vi "GoldenHour.vi"() -> ()   [LabVIEW 2019]
doc: "This example demonstrates how to read X, Y, and Z accelerations using the MMA8452 accelerometer."
uses:
  <vilib>/userdefined/High Color/IMAQdx.ctl
  System.Windows.Forms
  <vilib>/Utility/miscctls.llb/LVForegroundBackgroundColorsTypeDef.ctl
  <vilib>/Instr/_visa.llb/VISA Configure Serial Port (Instr).vi
  <vilib>/MakerHub/LINX/Public/Utilities/Open Serial.vi
  <vilib>/Utility/file.llb/Write Delimited Spreadsheet (DBL).vi
  <vilib>/Utility/file.llb/Read Delimited Spreadsheet (DBL).vi
  <vilib>/MakerHub/LINX/LMH-LINX.lvlib
  <vilib>/MakerHub/LINX/Public/Sensors/Accelerometer/MMA8452/MMA8452.lvlib
  <vilib>/vision/driver/NI_Vision_Acquisition_Software.lvlib
panel:
  in  "file path (dialog if empty)":path caption="파일 경로(비었을 경우 대화 상자 창)"
  in  "경로 2":path=path "C:/Users/suit9/Documents/카카오톡 받은 파일/inventors.csv"
  in  "경로":path=path "C:/Users/suit9/Documents/카카오톡 받은 파일/inventors - 복사본.csv"
  in  "A Port":refnum<visa-resource-name>
  in  "B Port":refnum<visa-resource-name>
  in  "Camera":T1
  in  "Grbl":refnum<visa-resource-name>="COM5"
  in  "B 설비 이상":bool
  in  "A 설비 이상":bool
  in  "B_stop":bool
  in  "A_stop":bool
  in  "CAM_stop":bool
  in  "P_stop":bool
  in  "I2C Channel 2":u8
  in  "CAM_Control":T2
  in  "Page_B":bool
  in  "Page_A":bool
  in  "Page_ALL":bool
  in  "distance(mm)":dbl=4.0
  out "Y_FFT 2":dbl[](graph)
  out "Z_FFT 2":dbl[](graph)
  in  "B_X_그림":path=path "C:/Users/suit9/Desktop/대회준비 모든파일/슈퍼이상.png"
  in  "A_X_그림":path=path "C:/Users/suit9/Desktop/대회준비 모든파일/정상.png"
  in  "B_Z":path=path "C:/Users/suit9/Desktop/대회준비 모든파일/엑셀모음/B_Z.csv"
  in  "B_Y":path=path "C:/Users/suit9/Desktop/대회준비 모든파일/엑셀모음/B_Y.csv"
  in  "B_X":path=path "C:/Users/suit9/Desktop/대회준비 모든파일/엑셀모음/B_X.csv"
  in  "A_Z":path=path "C:/Users/suit9/Desktop/대회준비 모든파일/엑셀모음/A_Z.csv"
  in  "A_Y":path=path "C:/Users/suit9/Desktop/대회준비 모든파일/엑셀모음/A_Y.csv"
  in  "A_X":path=path "C:/Users/suit9/Desktop/대회준비 모든파일/엑셀모음/A_X.csv"
  in  "dist(mm)":dbl
  in  "dist(mm) 2":dbl
  in  "A설비":dbl
  in  "B설비":dbl
  out "MoveString 5":string
  out "MoveString 4":string
  out "number 2":dbl format="%.2f"
  out "MoveString 3":string
  out "Version":string
  out "Connecting to":string
  in  "Send G-code":bool
  in  "Select G-code file":bool
  out "G-code list":string
  in  "Local-Home":bool
  in  "Pos Button":bool
  out "Local-Pos":cluster{"X":dbl, "Y":dbl, "Z":dbl}
  out "M-Pos":cluster{"X":dbl, "Y":dbl, "Z":dbl}
  in  "Machine-Home":bool
  in  "Send":bool
  in  "One line Command":string
  in  "SetLocal":bool
  out "Local Origin":cluster{"X":dbl, "Y":dbl, "Z":dbl}
  out "MoveString":string
  out "MoveString 2":string
  out "Command":string
  out "History":string
  out "Response":string
  in  "탭 컨트롤":enum32{"ALL", "A", "B"}(tab)
  out "특이사항":string="A설비 이상진동 다량발생 확인요함\n\n설비 이력\n\n# 이전 A설비 교체 : 2020-09-10\n\n# 이전 B설비 교체 : 2020-08-20\n\n\n"
  out "Boolean Rectangle 3":bool
  out "Boolean Rectangle":bool
  out "Time series 4":T3(graph)
  out "Time series 3":T3(graph)
  out "수명예측":dbl(knob) caption="Gauge" scale=0.1..100.0
  out "CAM":T4(plugin-control)
  out "all rows":dbl[][](array[numeric]) caption="NUM(A)    LOSS     THR        Vib"
  out "수명예측":dbl(knob) caption="Gauge" scale=0.0..100.0
  out "all rows 2":dbl[][](array[numeric]) caption="NUM(B)        LOSS      THR        Vib"
  out "수명예측":dbl(knob) caption="Gauge" scale=0.0..100.0
  out "문자열 2":string="A : 양호\n\nB : 약간불량, 장시간 운전 허용\n\nC : 불량, 단 시간 운전 허용\n\nD : 극도 불량, 허용불가"
  out "클러스터 6":cluster{"A":bool, "B":bool, "C":bool, "D":bool}
  out "FFT A":dbl[](graph)
  out "Time series A":T3(graph)
  out "CAM":T4(plugin-control)
  in  "PictureBox 5":refnum<k24>(container) caption="Anomaly Detection A"
  out "수명예측":dbl(knob) caption="Gauge" scale=0.1..100.0
  out "문자열":string="A : 양호\n\nB : 약간불량, 장시간 운전 허용\n\nC : 불량, 단 시간 운전 허용\n\nD : 극도 불량, 허용불가"
  out "클러스터 5":cluster{"A":bool, "B":bool, "C":bool, "D":bool}
  out "FFT_B":dbl[](graph)
  out "Time series B":T3(graph)
  out "CAM":T4(plugin-control)
  in  "PictureBox 2":refnum<k24>(container) caption="Anomaly Detection B"
  in  "I2C Channel":u8
  # "GOLDEN\n     Hour"
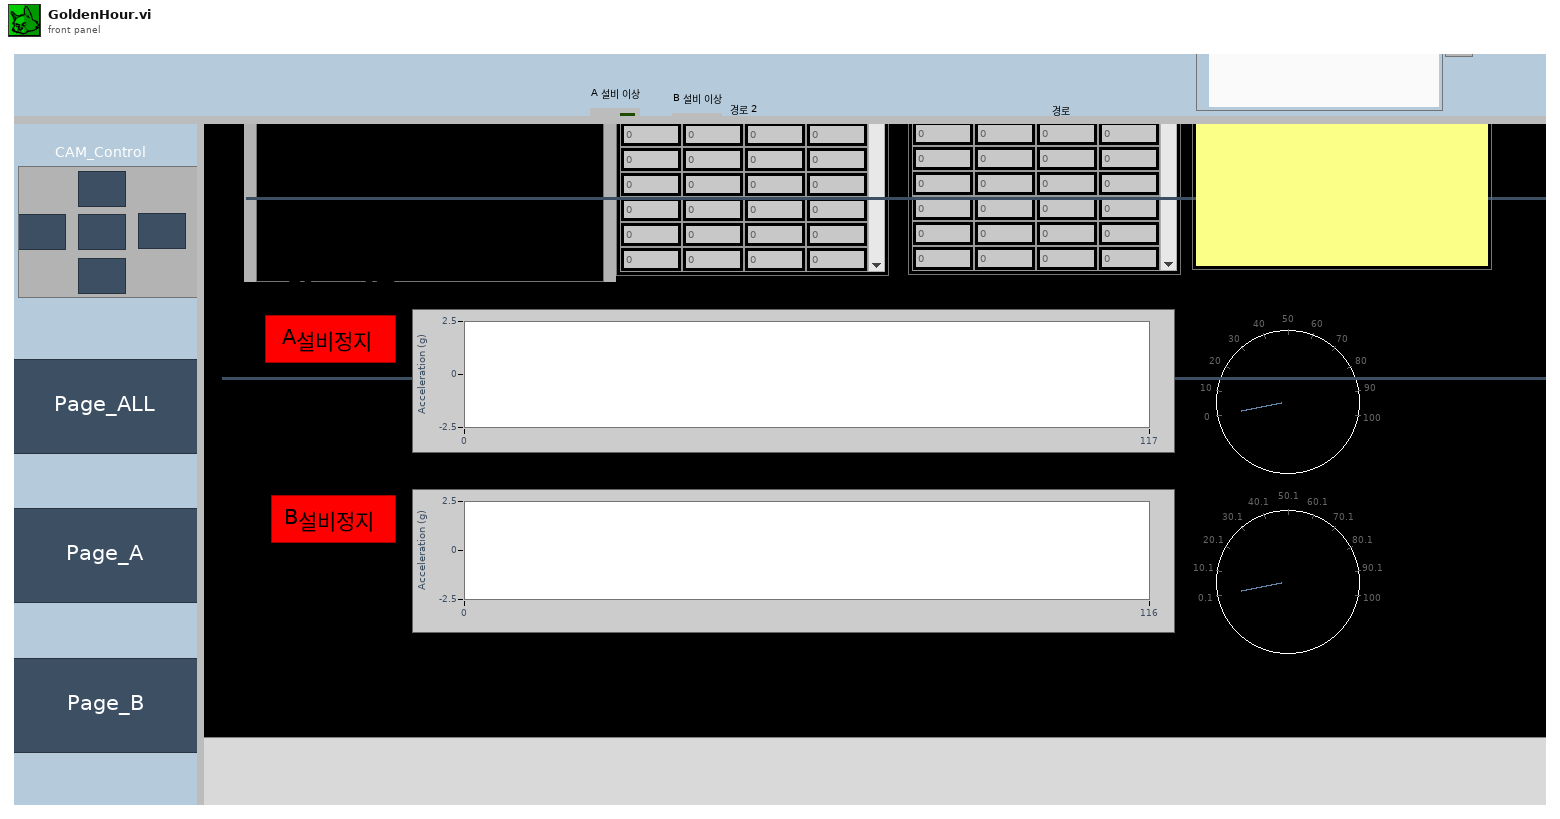
[diagram p1: front panel]
types:
  T1 = typedef "IMAQdx.ctl" = refnum<k21>
  T2 = cluster{"Back Button":bool, "Forward Button":bool, "Up Button":bool, "Down Button":bool, "Reset Button":bool}
  T3 = cluster{"X Axis":dbl, "Y Axis":dbl, "Z Axis":dbl}
  T4 = typedef "IMAQ Image.ctl" = refnum<image>
  T5 = cluster{"VISA resource name":refnum<visa-resource-name>, "baud rate":u32, "data bits":u16, "parity":u16, "stop bits":u16, "flow control":u16}
  T6 = typedef "LVForegroundBackgroundColorsTypeDef.ctl" = cluster{"Foreground Color":u32, "Background Color":u32}
  T7 = typedef "LMH-LINX.lvlib/LINX Ref.ctl" = cluster{"IO":T8, "Interface":T9, "LINX Device Config":T10}
  T8 = typedef "LMH-LINX.lvlib/Platform.ctl" = enum16{"Remote", "Local"}
  T9 = typedef "LMH-LINX.lvlib/Interface.ctl" = enum16{"Serial", "TCP"}
  T10 = typedef "LMH-LINX.lvlib/Device.lvlib/LINX Device Config.ctl" = cluster{"Interface":T9, "COM Port":refnum<visa-resource-name>, "TCP Configuration":T11, "Device Family":u8, "Device ID":u8, "Device Name":string, "TCP Ref":refnum<k5>, "Channels":T12}
  T11 = typedef "LMH-LINX.lvlib/Device.lvlib/TCP Config.ctl" = cluster{"IP Address":string, "Port":u16}
  T12 = typedef "LMH-LINX.lvlib/Channels.ctl" = cluster{"DI":u8[], "DO":u8[], "AI":u8[], "AO":u8[], "PWM":u8[], "QE":u8[], "UART":u8[], "I2C 2":u8[], "SPI":u8[], "CAN":u8[], "Servo":u8[], "AI Ref (V)":dbl, "AI Resolution (Bits)":u8, "AO Ref (V)":dbl, "AO Resolution (Bits)":u8}
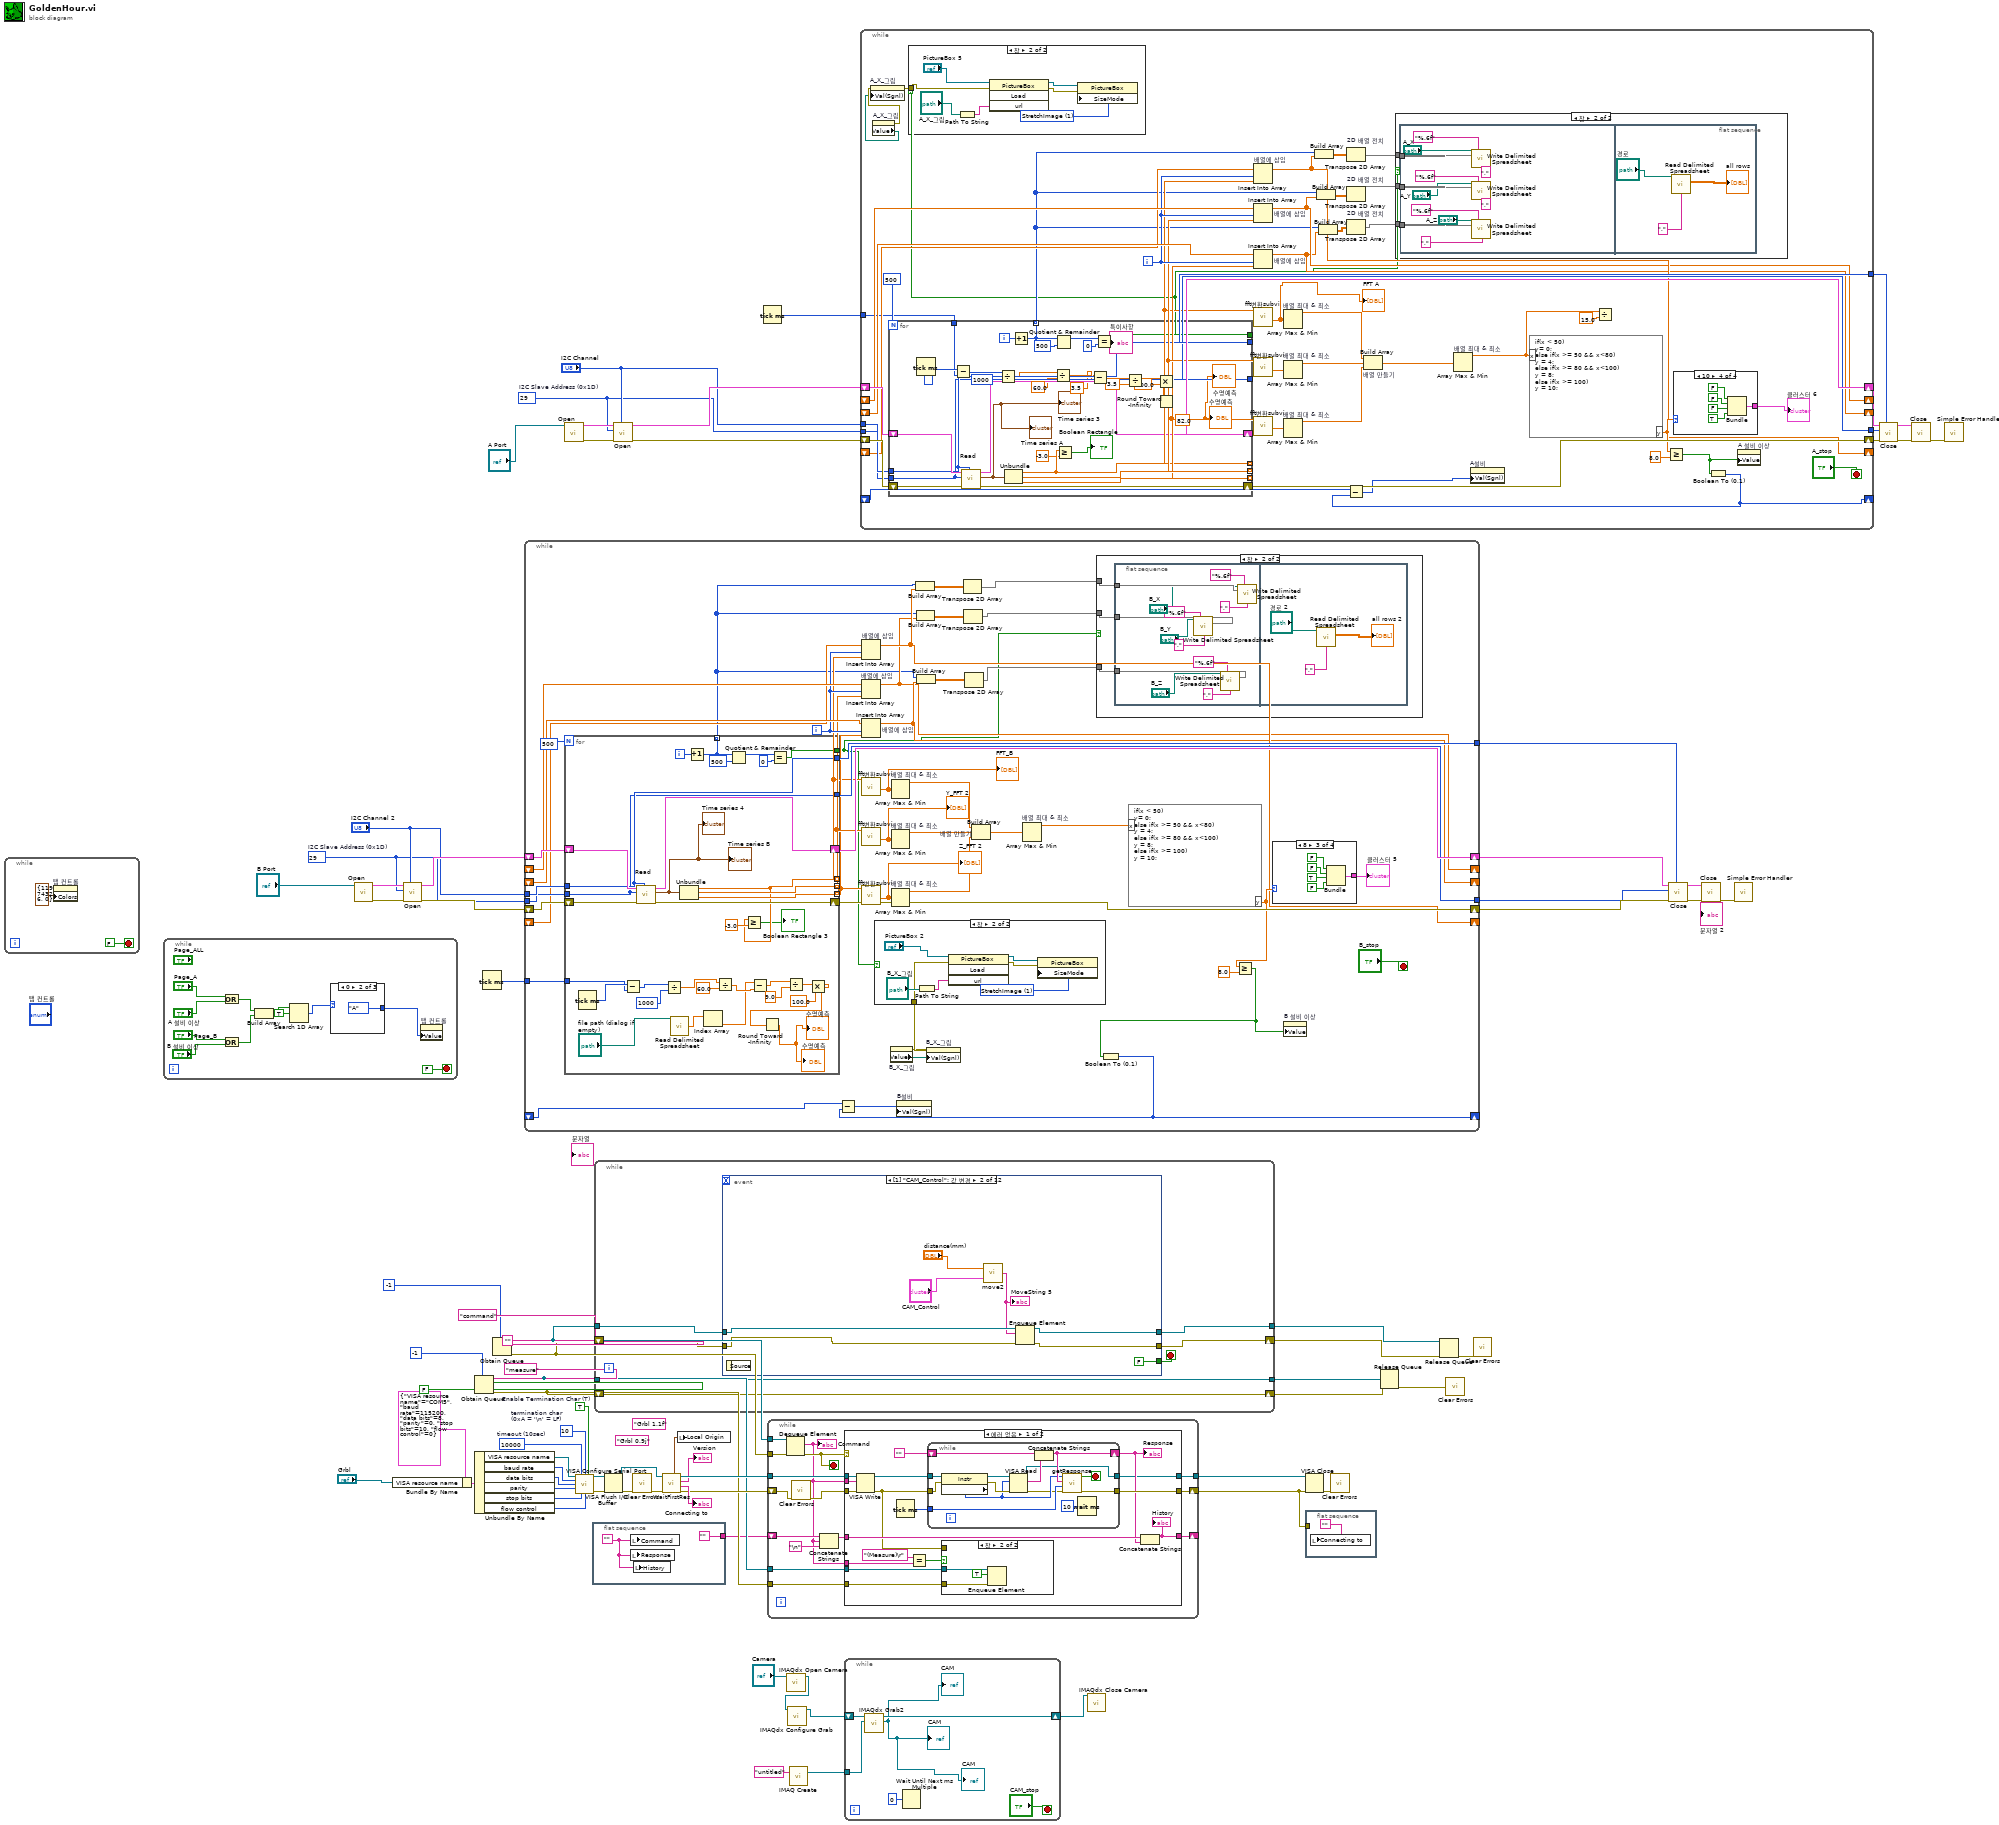
[diagram p0: block diagram]
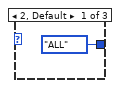
[diagram p2: hidden frame]
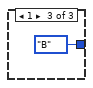
[diagram p3: hidden frame]
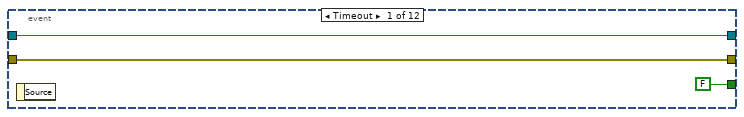
[diagram p4: hidden frame]
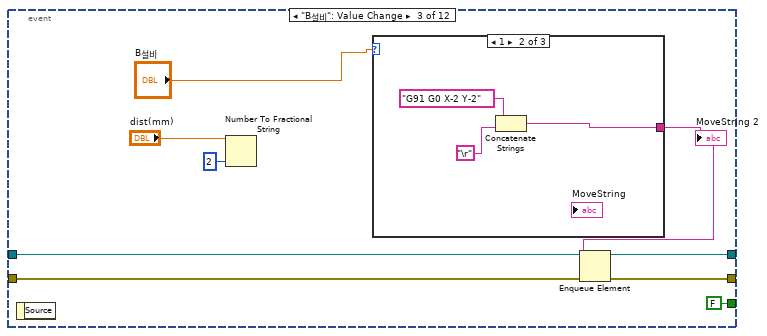
[diagram p5: hidden frame]
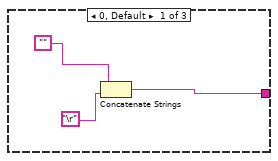
[diagram p6: hidden frame]
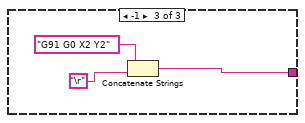
[diagram p7: hidden frame]
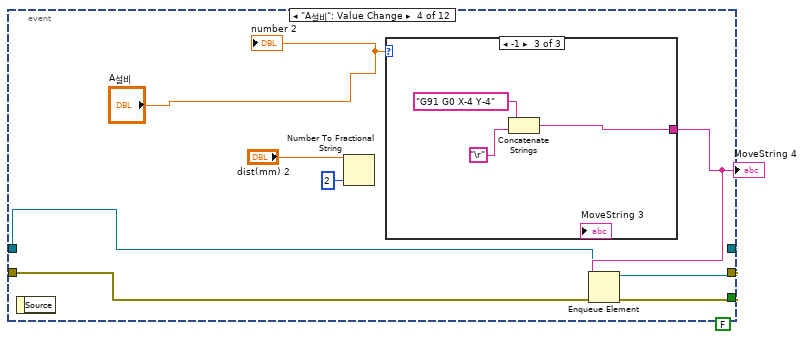
[diagram p8: hidden frame]
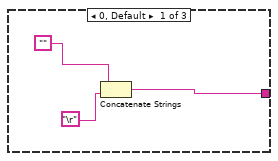
[diagram p9: hidden frame]
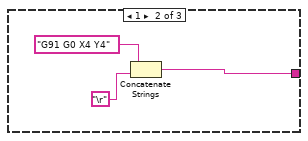
[diagram p10: hidden frame]
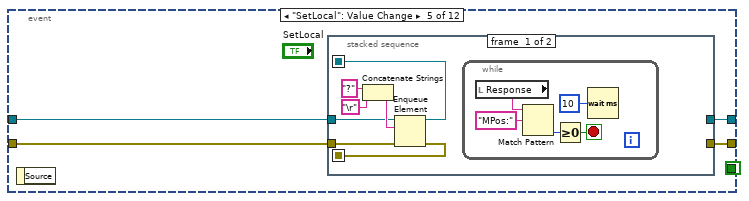
[diagram p11: hidden frame]
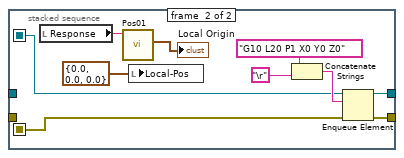
[diagram p12: hidden frame]
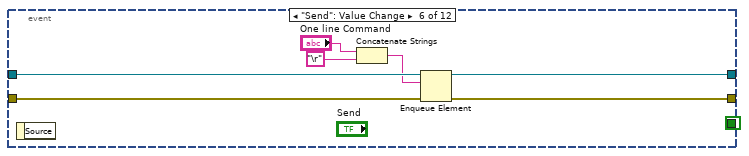
[diagram p13: hidden frame]
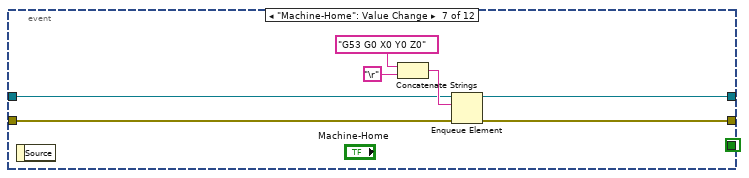
[diagram p14: hidden frame]
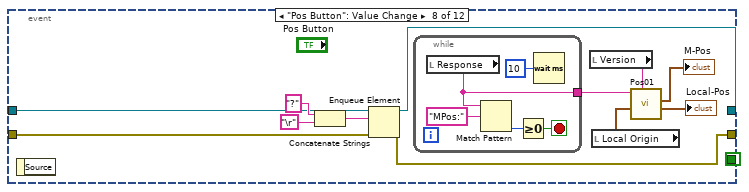
[diagram p15: hidden frame]
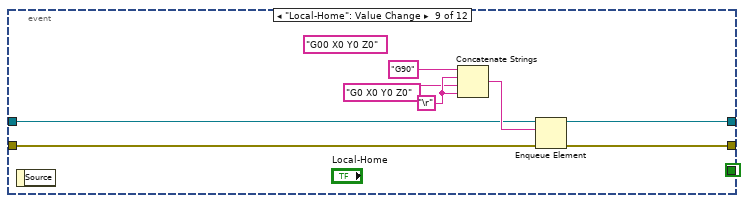
[diagram p16: hidden frame]
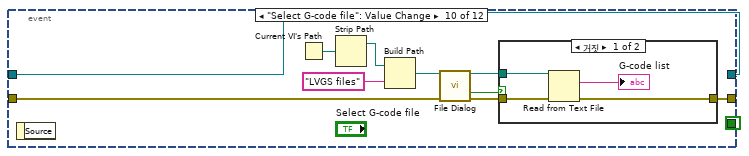
[diagram p17: hidden frame]
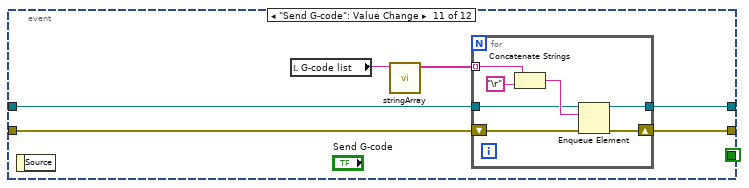
[diagram p19: hidden frame]
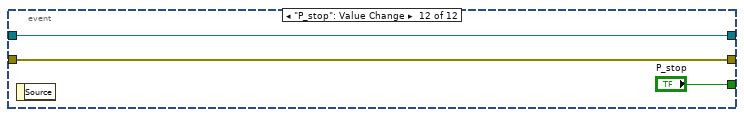
[diagram p20: hidden frame]
diagram:
  (unwired) "Grbl 1.1f" ("Version")
  (unwired) "Grbl 0.9j" ("Version")
  w31 = u8 10  # termination char (0xA = '\n' = LF)
  w42 = TRUE  # Enable Termination Char (T)
  w52 = u32 10000  # timeout (10sec)
  w60 = u8 29  # I2C Slave Address (0x1D)
  w73 = u8 29  # I2C Slave Address (0x1D)
  n1 = while {
    stop <- FALSE stop-if-true
    n2 = property on="탭 컨트롤" class="TabCtl (엄격한)"("Colors"=T6 {"Foreground Color"=11974326, "Background Color"=0} ("색")) -> ()  [unwired: 2 in, 2 out]
  }
  n3 = while {
    stop <- FALSE stop-if-true
    n4 = Or(x="Page_A", y="A 설비 이상") -> (x .or. y?=w87:bool)
    n5 = Or(x="Page_B", y="B 설비 이상") -> (x .or. y?=w86:bool)
    n6 = Build Array(w87, w86) -> (w85:bool[])
    n7 = Search 1D Array(1D array=w85, element=TRUE ("원소")) -> (index of element=w83:i32)  [unwired: 1 in]
    n8 = case shown="0" w83 {
      tunnel: [enum32{"ALL", "A", "B"}."ALL" ("탭 컨트롤") enum32{"ALL", "A", "B"}."A" ("탭 컨트롤") enum32{"ALL", "A", "B"}."B" ("탭 컨트롤")] -> w82
      frame 2, Default {
      }
      frame 0 {
      }
      frame 1 {
      }
    }
    n9 = property on="탭 컨트롤" class="TabCtl (엄격한)"("Value"=w82) -> ()  [unwired: 2 in, 2 out]
  }
  n10 = call-poly <vilib>:"Open.vi"("Serial Port"="B Port") -> ("Error Out"=w65:errorcluster, "LINX Resource"=w64:T7)  [unwired: 8 in, 1 out]
  n11 = Bundle By Name(cluster=T5 {"VISA resource name"="COM5", "baud rate"=115200, "data bits"=8, "parity"=0, "stop bits"=10, "flow control"=0} ("COM"), "VISA resource name"="Grbl") -> (w49:T5)
  n12 = call <vilib>:"Open.vi"("I2C Channel"="I2C Channel 2", "Error In"=w65, "I2C Slave Address (0x1D)"=w60, "LINX Ref"=w64) -> ("Error Out"=w62:errorcluster, "LINX Resource"=w63:T7)  [unwired: 6 in]
  n13 = Obtain Queue(max queue size (-1, unlimited)=-1, name (unnamed)="measure", element data type=FALSE) -> (queue out=w16:refnum<queue>, error out=w15:errorcluster)  [unwired: 2 in, 1 out]
  n14 = Unbundle By Name(w49) -> ("VISA resource name"=w48:refnum<visa-resource-name>, "baud rate"=w47:u32, "data bits"=w46:u16, "parity"=w45:u16, "stop bits"=w44:u16, "flow control"=w43:u16)
  n15 = Tick Count (ms)() -> (millisecond timer value=w1:u32)
  n16 = Obtain Queue(max queue size (-1, unlimited)=-1, name (unnamed)="command", element data type="") -> (queue out=w27:refnum<queue>, error out=w32:errorcluster)  [unwired: 2 in, 1 out]
  n17 = while {
    tunnel: "I2C Channel 2" -> [w139]
    tunnel: w60 -> [w138]
    tunnel: [w135] -> w54
    tunnel: [w134] -> w53
    shift-right: [w136] -> w57
    shift-left: w63 -> [w141]
    shift-right: [w137] -> w58
    shift-left: w62 -> [w140]
    shift-right: [w112] -> _
    shift-left: _ -> [w123]
    shift-right: [w105] -> _
    shift-left: _ -> [w132]
    shift-right: [w106] -> _
    shift-left: _ -> [w131]
    shift-right: [w114] -> _
    shift-left: _ -> [w115]
    tunnel: w1 -> [w99]
    i -> [w129]
    stop <- "B_stop" stop-if-true
    n18 = for {
      N: 500 -> [_]
      tunnel: w139 -> [w217]
      tunnel: w138 -> [w216]
      shift-right: [w219] -> w136
      shift-left: w141 -> [w218]
      shift-right: [w215] -> w137
      shift-left: w140 -> [w220]
      tunnel: [w217] -> w135
      tunnel: [w216] -> w134
      tunnel: [w205] -> w120 mode=indexing
      tunnel: [w213] -> w122 mode=indexing
      tunnel: [w214] -> w121 mode=indexing
      tunnel: [w209] -> w103
      tunnel: [w207] -> w104 mode=indexing
      tunnel: w99 -> [w201]
      i -> [w208]
      n19 = Tick Count (ms)() -> (millisecond timer value=w202:u32)
      n20 = Subtract(x=w202, y=w201) -> (x-y=w200:u32)
      n21 = call <vilib>:"Read.vi"("I2C Channel"=w217, "Error In"=w220, "I2C Slave Address (0x1D)"=w216, "LINX Resource in"=w218) -> ("Error Out"=w215:errorcluster, "Acceleration Data (g)"=w203:T3, "LINX Resource out"=w219:T7)  [unwired: 5 in]
      "Time series B" <- w203
      "Time series 4" <- w203
      n22 = Divide(x=w200, y=u32 1000) -> (x/y=w198:dbl)
      n23 = call-poly <vilib>:"Read Delimited Spreadsheet.vi"("file path (dialog if empty)"="file path (dialog if empty)") -> ("first row"=w188:dbl[])  [unwired: 9 in, 5 out]
      n24 = Unbundle(w203) -> ("X Axis"=w205:dbl, "Y Axis"=w213:dbl, "Z Axis"=w214:dbl)
      n25 = Increment(x=w208) -> (x+1=w207:i32)
      n26 = Index Array(array=w188) -> (element=w187:dbl)  [unwired: 1 in]
      n27 = Divide(x=w198, y=60.0) -> (x/y=w196:dbl)
      n28 = Quotient & Remainder(x=w207, y=500) -> (x-y*floor(x/y)=w210:i32)  [unwired: 1 out]
      n29 = Greater Or Equal?(x=w205, y=-3.0) -> (x >= y?=→"Boolean Rectangle 3":bool)
      n30 = Subtract(x=w187, y=w196) -> (x-y=w195:dbl)
      n31 = Equal?(x=w210, y=0) -> (x = y?=w209:bool)
      n32 = Divide(x=w195, y=9.0) -> (x/y=w193:dbl)
      n33 = Multiply(x=w193, y=100.0) -> (x*y=w191:dbl)
      n34 = Round Toward -Infinity(1:w191) -> (0:→"수명예측" →"수명예측":dbl)
    }
    n35 = Insert Into Array "배열에 삽입"(array=w123, index=w129, new element=w120) -> (w112:dbl[])
    n36 = Insert Into Array "배열에 삽입"(array=w132, index=w129, new element=w122) -> (w105:dbl[])
    n37 = Insert Into Array "배열에 삽입"(array=w131, index=w129, new element=w121) -> (w106:dbl[])
    n38 = call "fft변환subvi.vi"("배열"=w120) -> ("웨이브폼 그래프 4"=w102:dbl[])  [unwired: 7 in, 3 out]
    "FFT_B" <- w102
    n39 = call "fft변환subvi.vi"("배열"=w122) -> ("웨이브폼 그래프 4"=w101:dbl[])  [unwired: 7 in, 3 out]
    "Y_FFT 2" <- w101
    n40 = call "fft변환subvi.vi"("배열"=w121) -> ("웨이브폼 그래프 4"=w100:dbl[])  [unwired: 7 in, 3 out]
    "Z_FFT 2" <- w100
    n41 = property on="B_X_그림" class="Path"() -> (error out=w96:errorcluster, "Value"=w97:path)  [unwired: 2 in, 1 out]
    n42 = Array Max & Min "배열 최대 & 최소"(array=w102) -> (max value=w128:dbl)  [unwired: 3 out]
    n43 = Array Max & Min "배열 최대 & 최소"(array=w101) -> (max value=w127:dbl)  [unwired: 3 out]
    n44 = Array Max & Min "배열 최대 & 최소"(array=w100) -> (max value=w126:dbl)  [unwired: 3 out]
    n45 = Build Array(w104, w112) -> (w111:dbl[][])
    n46 = Build Array(w104, w105) -> (w110:dbl[][])
    n47 = Build Array(w104, w106) -> (w109:dbl[][])
    n48 = property on="B_X_그림" class="Path"(error in=w96, "Val(Sgnl)"=w97) -> (error out=w98:errorcluster)  [unwired: 1 in, 1 out]
    n49 = case shown="참" w103 {
      tunnel: w98 -> [_ w142]
      frame False {
      }
      frame True {
        w145 = 1 items=["Normal", "StretchImage", "AutoSize", "CenterImage", "Zoom"] ("SizeMode")
        n50 = Path To String(path="B_X_그림") -> (string=w148:string)
        n51 = invoke on="인보크 노드" class="PictureBox" method="Load"(reference="PictureBox 2", error in=w142, "url"=w148) -> (reference out=w147:refnum<k24>, error out=w146:errorcluster)  [unwired: 1 in, 2 out]
        n52 = property on="프로퍼티 노드" class="PictureBox"(reference=w147, error in=w146, "SizeMode"=w145) -> ()  [unwired: 2 out]
      }
    }
    n53 = Transpose 2D Array(2D array=w111) -> (transposed array=w130:dbl[][])
    n54 = Transpose 2D Array(2D array=w110) -> (transposed array=w108:dbl[][])
    n55 = Transpose 2D Array(2D array=w109) -> (transposed array=w107:dbl[][])
    n56 = Build Array "배열 만들기"(w128, w127, w126) -> (w125:dbl[])
    n57 = Array Max & Min "배열 최대 & 최소"(array=w125) -> (max value=w118:dbl)  [unwired: 3 out]
    n58 = case shown="참" w103 {
      tunnel: w130 -> [_ w171]
      tunnel: w108 -> [_ w170]
      tunnel: w107 -> [_ w169]
      frame False {
      }
      frame True {
        n59 = flat-sequence {
          tunnel: w171 -> [w183]
          tunnel: w170 -> [w176]
          tunnel: w169 -> [w175]
          frame #0 {
            n60 = call-poly <vilib>:"Write Delimited Spreadsheet.vi"("file path (dialog if empty)"="B_Y", "format (%.3f)"="%.6f", "2D data"=w176, "delimiter (\\t)"="," ("delimiter (\\t)")) -> ()  [unwired: 10 in, 2 out]
            n61 = call-poly <vilib>:"Write Delimited Spreadsheet.vi"("file path (dialog if empty)"="B_Z", "format (%.3f)"="%.6f", "2D data"=w175, "delimiter (\\t)"="," ("delimiter (\\t)")) -> ()  [unwired: 10 in, 2 out]
            n62 = call-poly <vilib>:"Write Delimited Spreadsheet.vi"("file path (dialog if empty)"="B_X", "format (%.3f)"="%.6f", "2D data"=w183, "delimiter (\\t)"="," ("delimiter (\\t)")) -> ()  [unwired: 10 in, 2 out]
          }
          frame #1 {
            n63 = call-poly <vilib>:"Read Delimited Spreadsheet.vi"("file path (dialog if empty)"="경로 2", "delimiter (\\t)"="," ("delimiter (\\t)")) -> ("all rows"=→"all rows 2":dbl[][])  [unwired: 8 in, 5 out]
          }
        }
      }
    }
    n64 = formula code="if(x < 50)\ny= 0;\nelse if(x >= 50 && x<80)\ny = 4;\nelse if(x >= 80 && x<100)\ny = 8;\nelse if(x >= 100)\ny = 10;"("x"=w118) -> ("y"=w117:dbl)
    n65 = Greater Or Equal?(x=w117, y=8.0) -> (x >= y?=w95:bool)
    n66 = Boolean To (0,1)(Boolean=w95) -> (0, 1=w114:i16)
    n67 = Subtract(x=w115, y=w114) -> (x-y=w113:i16)
    n68 = property on="B설비" class="DigNum (엄격한)"("Val(Sgnl)"=w113) -> ()  [unwired: 2 in, 2 out]
    n69 = case shown="8" w117 {
      tunnel: [w149 w154 w159 w164] -> w124
      frame 0, Default {
        n70 = Bundle(TRUE, FALSE, FALSE, FALSE) -> (w149:cluster{bool, bool, bool, bool})  [unwired: 1 in]
      }
      frame 4 {
        n71 = Bundle(FALSE, TRUE, FALSE, FALSE) -> (w154:cluster{bool, bool, bool, bool})  [unwired: 1 in]
      }
      frame 8 {
        n72 = Bundle(FALSE, FALSE, TRUE, FALSE) -> (w159:cluster{bool, bool, bool, bool})  [unwired: 1 in]
      }
      frame 10 {
        n73 = Bundle(FALSE, FALSE, FALSE, TRUE) -> (w164:cluster{bool, bool, bool, bool})  [unwired: 1 in]
      }
    }
    "클러스터 5" <- w124
    n74 = property on="B 설비 이상" class="Bool (엄격한)"("Value"=w95) -> ()  [unwired: 2 in, 2 out]
  }
  n75 = call-poly <vilib>:"Open.vi"("Serial Port"="A Port") -> ("Error Out"=w78:errorcluster, "LINX Resource"=w77:T7)  [unwired: 8 in, 1 out]
  n76 = call-poly "VISA Configure Serial Port"("VISA resource name"=w48, "timeout (10sec)"=w52, "termination char\n(0xA = '\\n' = LF)"=w31, "Enable Termination\nChar (T)"=w42, "baud rate (9600)"=w47, "data bits (8)"=w46, "parity (0:none)"=w45, "stop bits (10: 1 bit)"=w44, "flow control (0:none)"=w43) -> ("VISA resource name out"=w40:refnum<visa-resource-name>, "error out"=w41:errorcluster)  [unwired: 1 in, 4 out]
  n77 = flat-sequence {
    tunnel: [""] -> w14
    frame #0 {
      w222 = ""
      n78 = local write "Command"(w222) -> ()
      n79 = local write "Response"(w222) -> ()
      n80 = local write "History"(w222) -> ()
    }
  }
  n81 = while {
    tunnel: w27 -> [w228]
    shift-right: [w226] -> w35
    shift-left: w32 -> [w227]
    tunnel: [w225] -> w34
    tunnel: [w224] -> w18
    tunnel: w16 -> [w224]
    shift-right: [w223] -> w17
    shift-left: w15 -> [w223]
    stop <- w229 stop-if-true
    n82 = event shown="[1] \"CAM_Control\": 값 변경" {
      selector: _ -> [_ _ _ _ _ _ _ _ _ _ _ _]
      dyn-events: _ -> [_ _ _ _ _ _ _ _ _ _ _ _]
      timeout: _ -> [_ _ _ _ _ _ _ _ _ _ _ _]
      tunnel: [FALSE FALSE FALSE ("NewVal") _ FALSE ("stop") FALSE ("stop") FALSE ("stop") FALSE ("stop") FALSE ("stop") FALSE ("stop") FALSE ("stop") "P_stop"] -> w229
      tunnel: w228 -> [w230 w240 w248 w262 w277 w310 w311 w322 w341 w344 w365 w375]
      tunnel: w227 -> [w231 w239 w247 w261 w280 w309 w314 w325 w336 w345 w364 w374]
      tunnel: [w231 w237 w246 w259 w279 w303 w313 w320 w335 w347 w362 w374] -> w226
      tunnel: [w230 w238 w245 w260 w276 w304 w311 w322 w340 w344 w363 w375] -> w225
      event Timeout {
        n83 = event-data() -> ()  [unwired: 1 in, 1 out]
      }
      event "CAM_Control": Value Change {
        n84 = event-data() -> ()  [unwired: 1 in, 1 out]
        n85 = call "move2.vi"("CAM_Control"="CAM_Control", "dist(mm)"="distance(mm)") -> ("MoveString"=w235:string)
        "MoveString 5" <- w235
        n86 = Enqueue Element(queue=w240, element=w235, error in (no error)=w239) -> (queue out=w238:refnum<queue>, error out=w237:errorcluster)  [unwired: 1 in, 1 out]
      }
      event "B설비": Value Change {
        n87 = event-data() -> ()  [unwired: 1 in, 1 out]
        n88 = Number To Fractional String(number="dist(mm)", precision (6)=i16 2) -> ()  [unwired: 2 in, 1 out]
        n89 = case shown="1" "B설비" {
          tunnel: [w252 w254 w257] -> w241
          frame 0, Default {
            n90 = Concatenate Strings("", "\r") -> (w252:string)
          }
          frame 1 {
            n91 = Concatenate Strings("G91 G0 X-2 Y-2", "\r") -> (w254:string)
          }
          frame -1 {
            n92 = Concatenate Strings("G91 G0 X2 Y2", "\r") -> (w257:string)
          }
        }
        "MoveString 2" <- w241
        n93 = Enqueue Element(queue=w248, element=w241, error in (no error)=w247) -> (queue out=w245:refnum<queue>, error out=w246:errorcluster)  [unwired: 1 in, 1 out]
      }
      event "A설비": Value Change {
        (unwired) FALSE ("NewVal")
        n94 = event-data() -> ()  [unwired: 1 in, 1 out]
        n95 = Number To Fractional String(number="dist(mm) 2", precision (6)=i16 2) -> ()  [unwired: 2 in, 1 out]
        n96 = case shown="-1" "A설비" {
          tunnel: [w269 w271 w274] -> w264
          frame 0, Default {
            n97 = Concatenate Strings("", "\r") -> (w269:string)
          }
          frame 1 {
            n98 = Concatenate Strings("G91 G0 X4 Y4", "\r") -> (w271:string)
          }
          frame -1 {
            n99 = Concatenate Strings("G91 G0 X-4 Y-4", "\r") -> (w274:string)
          }
        }
        "MoveString 4" <- w264
        n100 = Enqueue Element(queue=w262, element=w264, error in (no error)=w261) -> (queue out=w260:refnum<queue>, error out=w259:errorcluster)  [unwired: 1 in, 1 out]
        "number 2" <- "A설비"
      }
      event "SetLocal": Value Change {
        n101 = event-data() -> ()  [unwired: 1 in, 1 out]
        n102 = stacked-sequence {
          seq-local: [w282 _] -> [_ w296]
          seq-local: [w281 _] -> [_ w297]
          tunnel: w280 -> [w283 _]
          tunnel: [_ w298] -> w279
          tunnel: w277 -> [w284 _]
          tunnel: [_ w299] -> w276
          frame #0 {
            n103 = Concatenate Strings("?" ("Command 2"), "\r") -> (w285:string)
            n104 = Enqueue Element(queue=w284, element=w285, error in (no error)=w283) -> (queue out=w282:refnum<queue>, error out=w281:errorcluster)  [unwired: 1 in, 1 out]
            n105 = while {
              stop <- w290 stop-if-true
              n106 = local read "Response"() -> (w289:string)
              n107 = Match Pattern(string=w289, regular expression="MPos:") -> (offset past match=w291:i32)  [unwired: 1 in, 3 out]
              n108 = Greater Or Equal To 0?(x=w291) -> (x >= 0?=w290:bool)
              n109 = Wait (ms)(milliseconds to wait=u32 10) -> ()  [unwired: 1 out]
            }
          }
          frame #1 {
            n110 = local read "Response"() -> (w295:string)
            n111 = call "Pos01.vi"("String"=w295) -> ("M-Pos"=→"Local Origin":cluster{"X":dbl, "Y":dbl, "Z":dbl})  [unwired: 9 in, 1 out]
            n112 = local write "Local-Pos"(cluster{"X":dbl, "Y":dbl, "Z":dbl} {"X"=0.0, "Y"=0.0, "Z"=0.0} ("Local-Pos")) -> ()
            n113 = Concatenate Strings("G10 L20 P1 X0 Y0 Z0" ("format string"), "\r") -> (w301:string)
            n114 = Enqueue Element(queue=w296, element=w301, error in (no error)=w297) -> (queue out=w299:refnum<queue>, error out=w298:errorcluster)  [unwired: 1 in, 1 out]
          }
        }
      }
      event "Send": Value Change {
        n115 = event-data() -> ()  [unwired: 1 in, 1 out]
        n116 = Concatenate Strings("One line Command", "\r") -> (w305:string)
        n117 = Enqueue Element(queue=w310, element=w305, error in (no error)=w309) -> (queue out=w304:refnum<queue>, error out=w303:errorcluster)  [unwired: 1 in, 1 out]
      }
      event "Machine-Home": Value Change {
        n118 = event-data() -> ()  [unwired: 1 in, 1 out]
        n119 = Concatenate Strings("G53 G0 X0 Y0 Z0" ("Command 2"), "\r") -> (w315:string)
        n120 = Enqueue Element(queue=w311, element=w315, error in (no error)=w314) -> (error out=w313:errorcluster)  [unwired: 1 in, 2 out]
      }
      event "Pos Button": Value Change {
        n121 = event-data() -> ()  [unwired: 1 in, 1 out]
        n122 = Concatenate Strings("?" ("Command 2"), "\r") -> (w326:string)
        n123 = Enqueue Element(queue=w322, element=w326, error in (no error)=w325) -> (error out=w320:errorcluster)  [unwired: 1 in, 2 out]
        n124 = while {
          tunnel: [w330] -> w321
          stop <- w331 stop-if-true
          n125 = local read "Response"() -> (w330:string)
          n126 = Match Pattern(string=w330, regular expression="MPos:") -> (offset past match=w332:i32)  [unwired: 1 in, 3 out]
          n127 = Greater Or Equal To 0?(x=w332) -> (x >= 0?=w331:bool)
          n128 = Wait (ms)(milliseconds to wait=u32 10) -> ()  [unwired: 1 out]
        }
        n129 = local read "Version"() -> (w318:string)
        n130 = local read "Local Origin"() -> (w319:cluster{"X":dbl, "Y":dbl, "Z":dbl})
        n131 = call "Pos01.vi"("Version"=w318, "Local Origin"=w319, "String"=w321) -> ("W-Pos"=→"Local-Pos":cluster{"X":dbl, "Y":dbl, "Z":dbl}, "M-Pos"=→"M-Pos":cluster{"X":dbl, "Y":dbl, "Z":dbl})  [unwired: 7 in]
      }
      event "Local-Home": Value Change {
        (unwired) "G00 X0 Y0 Z0" ("Command 2")
        w339 = "\r"
        n132 = event-data() -> ()  [unwired: 1 in, 1 out]
        n133 = Concatenate Strings("G90" ("Command 2"), w339, "G0 X0 Y0 Z0" ("Command 2"), w339) -> (w342:string)
        n134 = Enqueue Element(queue=w341, element=w342, error in (no error)=w336) -> (queue out=w340:refnum<queue>, error out=w335:errorcluster)  [unwired: 1 in, 1 out]
      }
      event "Select G-code file": Value Change {
        n135 = event-data() -> ()  [unwired: 1 in, 1 out]
        n136 = Current VI's Path() -> (path=w354:path)
        n137 = Strip Path(path=w354) -> (stripped path=w353:path)  [unwired: 1 out]
        n138 = Build Path(base path=w353, name or relative path="LVGS files") -> (appended path=w351:path)
        n139 = call "File Dialog"("start path"=w351, "error in"=w345) -> ("selected path"=w349:path, "cancelled"=w350:bool, "error out"=w348:errorcluster)  [unwired: 10 in, 1 out]
        n140 = case shown="거짓" w350 {
          tunnel: w349 -> [w358 _]
          tunnel: w348 -> [w356 w359]
          tunnel: [w355 w359] -> w347
          frame False {
            n141 = Read from Text File(file (use dialog)=w358, error in=w356) -> (text=→"G-code list":string, error out=w355:errorcluster)  [unwired: 2 in, 2 out]
          }
          frame True {
          }
        }
      }
      event "Send G-code": Value Change {
        n142 = event-data() -> ()  [unwired: 1 in, 1 out]
        n143 = local read "G-code list"() -> (w366:string)
        n144 = call "stringArray.vi"("CNC strings"=w366) -> ("stringArray"=w361:string[])  [unwired: 10 in]
        n145 = for {
          tunnel: w365 -> [w371]
          tunnel: [w369] -> w363
          shift-right: [w368] -> w362
          shift-left: w364 -> [w370]
          tunnel: w361 -> [w367] mode=indexing
          n146 = Concatenate Strings(w367, "\r") -> (w372:string)
          n147 = Enqueue Element(queue=w371, element=w372, error in (no error)=w370) -> (queue out=w369:refnum<queue>, error out=w368:errorcluster)  [unwired: 1 in, 1 out]
        }
      }
      event "P_stop": Value Change {
        n148 = event-data() -> ()  [unwired: 1 in, 1 out]
      }
    }
  }
  n149 = VISA Flush I/O Buffer(VISA resource name=w40, error in (no error)=w41) -> (VISA resource name out=w30:refnum<visa-resource-name>, error out=w26:errorcluster)  [unwired: 1 in]
  n150 = call <vilib>:"Open.vi"("I2C Channel"="I2C Channel", "Error In"=w78, "I2C Slave Address (0x1D)"=w73, "LINX Ref"=w77) -> ("Error Out"=w75:errorcluster, "LINX Resource"=w76:T7)  [unwired: 6 in]
  n151 = call <vilib>:"Clear Errors.vi"("error in (no error)"=w26) -> ("error out"=w25:errorcluster)  [unwired: 5 in, 1 out]
  n152 = call "WaitFirstRes.vi"("error in (no error)"=w25, "VISA in"=w30) -> ("error out"=w24:errorcluster, "String"=→"Connecting to":string, "Version"=→"Version":string, "VISA out"=w29:refnum<visa-resource-name>, "Local Origin"=w12:cluster{"X":dbl, "Y":dbl, "Z":dbl})  [unwired: 4 in, 1 out]
  n153 = local write "Local Origin"(w12) -> ()
  n154 = Tick Count (ms)() -> (millisecond timer value=w2:u32)
  n155 = while {
    tunnel: w29 -> [w390]
    shift-right: [w385] -> w23
    shift-left: w24 -> [w382]
    tunnel: [w386] -> w51
    shift-right: [w387] -> _
    shift-left: w14 -> [w389]
    tunnel: w27 -> [w391]
    tunnel: w32 -> [w384]
    tunnel: w16 -> [w378]
    tunnel: w15 -> [w377]
    stop <- w383 stop-if-true
    n156 = Dequeue Element(queue=w391, error in (no error)=w384) -> (element=w379:string, error out=w383:errorcluster)  [unwired: 1 in, 2 out]
    "Command" <- w379
    n157 = call <vilib>:"Clear Errors.vi"("error in (no error)"=w382) -> ("error out"=w381:errorcluster)  [unwired: 5 in, 1 out]
    n158 = Concatenate Strings(w389, w379, "\n") -> (w388:string)
    n159 = case shown="에러 없음" w383 {
      tunnel: w390 -> [w408 w427]
      tunnel: w379 -> [w406 _]
      tunnel: w388 -> [w403 w426]
      tunnel: [w402 w426] -> w387
      tunnel: [w392 w427] -> w386
      tunnel: [w405 w428] -> w385
      tunnel: w381 -> [w404 w428]
      tunnel: w379 -> [w393 _]
      tunnel: w378 -> [w396 _]
      tunnel: w377 -> [w395 _]
      frame No Error {
        n160 = VISA Write(VISA resource name=w408, write buffer=w406, error in (no error)=w404) -> (VISA resource name out=w407:refnum<visa-resource-name>, error out=w394:errorcluster)  [unwired: 1 out]
        n161 = Tick Count (ms)() -> (millisecond timer value=w399:u32)
        n162 = Equal?(x="(Measure)\r" ("y"), y=w393) -> (x = y?=w397:bool)
        n163 = while {
          tunnel: w407 -> [w425]
          tunnel: w394 -> [w413]
          shift-right: [w420] -> w400
          shift-left: "" -> [w422]
          tunnel: [w412] -> w392
          tunnel: [w415] -> w405
          tunnel: w399 -> [w419]
          stop <- w417 stop-if-true
          n164 = property class="Instr"(reference=w425, error in=w413) -> (reference out=w423:refnum<visa-resource-name>, error out=w424:errorcluster, "Serial Settings:Number of Bytes at Serial Port"=w418:u32)
          n165 = VISA Read(VISA resource name=w423, byte count=w418, error in (no error)=w424) -> (VISA resource name out=w412:refnum<visa-resource-name>, read buffer=w421:string, error out=w416:errorcluster)  [unwired: 1 out]
          n166 = Concatenate Strings(w422, w421) -> (w420:string)
          n167 = call "getResponse.vi"("error in (no error)"=w416, "ST"=w419, "string"=w420, "Bytes at Serial Port"=w418) -> ("error out"=w415:errorcluster, "done"=w417:bool)  [unwired: 5 in, 1 out]
          n168 = Wait (ms)(milliseconds to wait=u32 10) -> ()  [unwired: 1 out]
        }
        "Response" <- w400
        n169 = case shown="참" w397 {
          tunnel: w396 -> [_ w411]
          tunnel: w395 -> [_ w410]
          tunnel: w394 -> [_ _]
          frame False {
          }
          frame True {
            n170 = Enqueue Element(queue=w411, element=TRUE, error in (no error)=w410) -> ()  [unwired: 1 in, 3 out]
          }
        }
        n171 = Concatenate Strings(w403, w400) -> (w402:string)
        "History" <- w402
      }
      frame Error {
      }
    }
  }
  n172 = call <vilib>:"IMAQdx Open Camera.vi"("Session In"="Camera") -> ("Session Out"=w9:T1)  [unwired: 9 in, 1 out]
  n173 = call <vilib>:"IMAQdx Configure Grab.vi"("Session In"=w9) -> ("Session Out"=w8:T1)  [unwired: 9 in, 1 out]
  n174 = call "IMAQ Create"("Image Name"="untitled") -> ("New Image"=w7:T4)  [unwired: 4 in, 1 out]
  n175 = while {
    tunnel: w7 -> [w433]
    shift-right: [w432] -> w5
    shift-left: w8 -> [w434]
    stop <- "CAM_stop" stop-if-true
    n176 = call <vilib>:"IMAQdx Grab2.vi"("Image In"=w433, "Session In"=w434) -> ("Image Out"=→"CAM" →"CAM" →"CAM":T4, "Session Out"=w432:T1)  [unwired: 6 in, 2 out]
    n177 = Wait Until Next ms Multiple(millisecond multiple=u32 0 ("ms 배수")) -> ()  [unwired: 1 out]
  }
  n178 = while {
    tunnel: "I2C Channel" -> [w480]
    tunnel: w73 -> [w479]
    tunnel: [w476] -> w67
    tunnel: [w475] -> w66
    shift-right: [w477] -> w70
    shift-left: w76 -> [w482]
    shift-right: [w478] -> w71
    shift-left: w75 -> [w481]
    shift-right: [w451] -> _
    shift-left: _ -> [w465]
    shift-right: [w450] -> _
    shift-left: _ -> [w473]
    shift-right: [w449] -> _
    shift-left: _ -> [w472]
    shift-right: [w456] -> _
    shift-left: _ -> [w455]
    tunnel: w2 -> [w439]
    i -> [w470]
    stop <- "A_stop" stop-if-true
    n179 = property on="A_X_그림" class="Path"() -> (error out=w437:errorcluster, "Value"=w436:path)  [unwired: 2 in, 1 out]
    n180 = property on="A_X_그림" class="Path"(error in=w437, "Val(Sgnl)"=w436) -> (error out=w438:errorcluster)  [unwired: 1 in, 1 out]
    n181 = for {
      N: 500 -> [_]
      tunnel: w480 -> [w556]
      tunnel: w479 -> [w555]
      shift-right: [w558] -> w477
      shift-left: w482 -> [w557]
      shift-right: [w554] -> w478
      shift-left: w481 -> [w559]
      tunnel: [w556] -> w476
      tunnel: [w555] -> w475
      tunnel: [w545] -> w460 mode=indexing
      tunnel: [w552] -> w464 mode=indexing
      tunnel: [w553] -> w463 mode=indexing
      tunnel: [w548] -> w444
      tunnel: [w546] -> w448 mode=indexing
      tunnel: w439 -> [w529]
      i -> [w547]
      w528 = 82.0 ("수명예측")
      n182 = Tick Count (ms)() -> (millisecond timer value=w541:u32)
      n183 = Subtract(x=w541, y=w529) -> (x-y=w540:u32)
      n184 = call <vilib>:"Read.vi"("I2C Channel"=w556, "Error In"=w559, "I2C Slave Address (0x1D)"=w555, "LINX Resource in"=w557) -> ("Error Out"=w554:errorcluster, "Acceleration Data (g)"=w542:T3, "LINX Resource out"=w558:T7)  [unwired: 5 in]
      "Time series A" <- w542
      "Time series 3" <- w542
      n185 = Divide(x=w540, y=u32 1000) -> (x/y=w538:dbl)
      n186 = Unbundle(w542) -> ("X Axis"=w545:dbl, "Y Axis"=w552:dbl, "Z Axis"=w553:dbl)
      n187 = Increment(x=w547) -> (x+1=w546:i32)
      n188 = Divide(x=w538, y=60.0) -> (x/y=w531:dbl)
      n189 = Quotient & Remainder(x=w546, y=500) -> (x-y*floor(x/y)=w549:i32)  [unwired: 1 out]
      n190 = Greater Or Equal?(x=w545, y=-3.0) -> (x >= y?=→"Boolean Rectangle":bool)
      n191 = Subtract(x=3.5 ("y"), y=w531) -> (x-y=w536:dbl)
      n192 = Equal?(x=w549, y=0) -> (x = y?=w548:bool)
      n193 = Divide(x=w536, y=3.5) -> (x/y=w534:dbl)
      n194 = Multiply(x=w534, y=100.0) -> (x*y=w532:dbl)
      n195 = Round Toward -Infinity(1:w532) -> ()  [unwired: 1 out]
      "수명예측" <- w528
      "수명예측" <- w528
    }
    n196 = case shown="참" w444 {
      tunnel: w438 -> [_ w483]
      frame False {
      }
      frame True {
        w486 = 1 items=["Normal", "StretchImage", "AutoSize", "CenterImage", "Zoom"] ("SizeMode")
        n197 = Path To String(path="A_X_그림") -> (string=w489:string)
        n198 = invoke on="인보크 노드" class="PictureBox" method="Load"(reference="PictureBox 5", error in=w483, "url"=w489) -> (reference out=w488:refnum<k24>, error out=w487:errorcluster)  [unwired: 1 in, 2 out]
        n199 = property on="프로퍼티 노드" class="PictureBox"(reference=w488, error in=w487, "SizeMode"=w486) -> ()  [unwired: 2 out]
      }
    }
    n200 = Insert Into Array "배열에 삽입"(array=w465, index=w470, new element=w460) -> (w451:dbl[])
    n201 = Insert Into Array "배열에 삽입"(array=w473, index=w470, new element=w464) -> (w450:dbl[])
    n202 = Insert Into Array "배열에 삽입"(array=w472, index=w470, new element=w463) -> (w449:dbl[])
    n203 = call "fft변환subvi.vi"("배열"=w460) -> ("웨이브폼 그래프 4"=w441:dbl[])  [unwired: 7 in, 3 out]
    "FFT A" <- w441
    n204 = call "fft변환subvi.vi"("배열"=w464) -> ("웨이브폼 그래프 4"=w443:dbl[])  [unwired: 7 in, 3 out]
    n205 = call "fft변환subvi.vi"("배열"=w463) -> ("웨이브폼 그래프 4"=w442:dbl[])  [unwired: 7 in, 3 out]
    n206 = Array Max & Min "배열 최대 & 최소"(array=w441) -> (max value=w469:dbl)  [unwired: 3 out]
    n207 = Array Max & Min "배열 최대 & 최소"(array=w443) -> (max value=w468:dbl)  [unwired: 3 out]
    n208 = Array Max & Min "배열 최대 & 최소"(array=w442) -> (max value=w467:dbl)  [unwired: 3 out]
    n209 = Build Array(w448, w451) -> (w447:dbl[][])
    n210 = Build Array(w448, w450) -> (w446:dbl[][])
    n211 = Build Array(w448, w449) -> (w445:dbl[][])
    n212 = Transpose 2D Array "2D 배열 전치"(2D array=w447) -> (transposed array=w471:dbl[][])
    n213 = Transpose 2D Array "2D 배열 전치"(2D array=w446) -> (transposed array=w453:dbl[][])
    n214 = Transpose 2D Array "2D 배열 전치"(2D array=w445) -> (transposed array=w452:dbl[][])
    n215 = Build Array "배열 만들기"(w469, w468, w467) -> (w466:dbl[])
    n216 = case shown="참" w444 {
      tunnel: w471 -> [_ w512]
      tunnel: w453 -> [_ w511]
      tunnel: w452 -> [_ w510]
      frame False {
      }
      frame True {
        n217 = flat-sequence {
          tunnel: w512 -> [w524]
          tunnel: w511 -> [w517]
          tunnel: w510 -> [w516]
          frame #0 {
            n218 = call-poly <vilib>:"Write Delimited Spreadsheet.vi"("file path (dialog if empty)"="A_X", "format (%.3f)"="%.6f", "2D data"=w524, "delimiter (\\t)"="," ("delimiter (\\t)")) -> ()  [unwired: 10 in, 2 out]
            n219 = call-poly <vilib>:"Write Delimited Spreadsheet.vi"("file path (dialog if empty)"="A_Y", "format (%.3f)"="%.6f", "2D data"=w517, "delimiter (\\t)"="," ("delimiter (\\t)")) -> ()  [unwired: 10 in, 2 out]
            n220 = call-poly <vilib>:"Write Delimited Spreadsheet.vi"("file path (dialog if empty)"="A_Z", "format (%.3f)"="%.6f", "2D data"=w516, "delimiter (\\t)"="," ("delimiter (\\t)")) -> ()  [unwired: 10 in, 2 out]
          }
          frame #1 {
            n221 = call-poly <vilib>:"Read Delimited Spreadsheet.vi"("file path (dialog if empty)"="경로", "delimiter (\\t)"="," ("delimiter (\\t)")) -> ("all rows"=→"all rows":dbl[][])  [unwired: 8 in, 5 out]
          }
        }
      }
    }
    n222 = Array Max & Min "배열 최대 & 최소"(array=w466) -> (max value=w462:dbl)  [unwired: 3 out]
    n223 = formula code="if(x < 50)\ny= 0;\nelse if(x >= 50 && x<80)\ny = 4;\nelse if(x >= 80 && x<100)\ny = 8;\nelse if(x >= 100)\ny = 10;"("x"=w462) -> ("y"=w457:dbl)
    n224 = Divide(x=w462, y=15.0) -> ()  [unwired: 1 out]
    n225 = Greater Or Equal?(x=w457, y=8.0) -> (x >= y?=w435:bool)
    n226 = case shown="10" w457 {
      tunnel: [w490 w495 w500 w505] -> w440
      frame 0, Default {
        n227 = Bundle(TRUE, FALSE, FALSE, FALSE) -> (w490:cluster{bool, bool, bool, bool})  [unwired: 1 in]
      }
      frame 4 {
        n228 = Bundle(FALSE, TRUE, FALSE, FALSE) -> (w495:cluster{bool, bool, bool, bool})  [unwired: 1 in]
      }
      frame 8 {
        n229 = Bundle(FALSE, FALSE, TRUE, FALSE) -> (w500:cluster{bool, bool, bool, bool})  [unwired: 1 in]
      }
      frame 10 {
        n230 = Bundle(FALSE, FALSE, FALSE, TRUE) -> (w505:cluster{bool, bool, bool, bool})  [unwired: 1 in]
      }
    }
    "클러스터 6" <- w440
    n231 = Boolean To (0,1)(Boolean=w435) -> (0, 1=w456:i16)
    n232 = Subtract(x=w455, y=w456) -> (x-y=w454:i16)
    n233 = property on="A설비" class="DigNum (엄격한)"("Val(Sgnl)"=w454) -> ()  [unwired: 2 in, 2 out]
    n234 = property on="A 설비 이상" class="Bool (엄격한)"("Value"=w435) -> ()  [unwired: 2 in, 2 out]
  }
  n235 = call <vilib>:"IMAQdx Close Camera.vi"("Session In"=w5) -> ()  [unwired: 10 in, 1 out]
  n236 = VISA Close(VISA resource name=w51, error in (no error)=w23) -> (error out=w39:errorcluster)
  n237 = flat-sequence {
    tunnel: w23 -> [_]
    frame #0 {
      n238 = local write "Connecting to"("") -> ()
    }
  }
  n239 = call <vilib>:"Clear Errors.vi"("error in (no error)"=w39) -> ()  [unwired: 5 in, 2 out]
  n240 = Release Queue(queue=w18, error in (no error)=w17) -> (error out=w19:errorcluster)  [unwired: 1 in, 2 out]
  n241 = Release Queue(queue=w34, error in (no error)=w35) -> (error out=w33:errorcluster)  [unwired: 1 in, 2 out]
  n242 = call <vilib>:"Clear Errors.vi"("error in (no error)"=w19) -> ()  [unwired: 5 in, 2 out]
  n243 = call <vilib>:"Clear Errors.vi"("error in (no error)"=w33) -> ()  [unwired: 5 in, 2 out]
  n244 = call <vilib>:"Close.vi"("I2C Channel (0)"=w54, "Error In"=w58, "I2C Slave Address (0)"=w53, "LINX Resource"=w57) -> ("Error Out"=w55:errorcluster, "LINX Resource"=w56:T7)  [unwired: 6 in]
  n245 = call <vilib>:"Close.vi"("Error In"=w55, "LINX Resource"=w56) -> ("Error Out"=w59:errorcluster)  [unwired: 9 in]
  n246 = call <vilib>:"Simple Error Handler.vi"("error in (no error)"=w59) -> ()  [unwired: 4 in, 5 out]
  n247 = call <vilib>:"Close.vi"("I2C Channel (0)"=w67, "Error In"=w71, "I2C Slave Address (0)"=w66, "LINX Resource"=w70) -> ("Error Out"=w68:errorcluster, "LINX Resource"=w69:T7)  [unwired: 6 in]
  n248 = call <vilib>:"Close.vi"("Error In"=w68, "LINX Resource"=w69) -> ("Error Out"=w72:errorcluster)  [unwired: 9 in]
  n249 = call <vilib>:"Simple Error Handler.vi"("error in (no error)"=w72) -> ()  [unwired: 4 in, 5 out]
